vi "Check and update pretomo counters.vi"(8 "error in (no error)":errorcluster, 11 "Tomo in":refnum<class "Tomo.lvclass">) -> (0 "error out":errorcluster, 1 "continue stack?":bool, 2 "continue acquiring?":bool, 3 "Tomo out":refnum<class "Tomo.lvclass">)   [LabVIEW 2012, in "Tomo.lvclass"]
uses:
  Tomo.lvclass
  Tomo.lvclass/Tomo.ctl
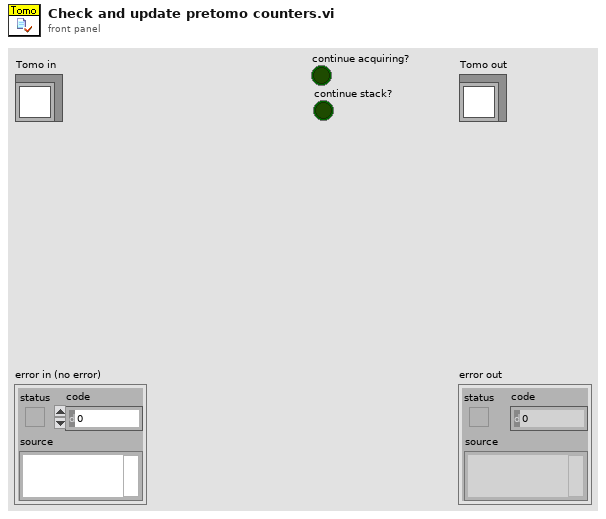
[diagram p1: front panel]
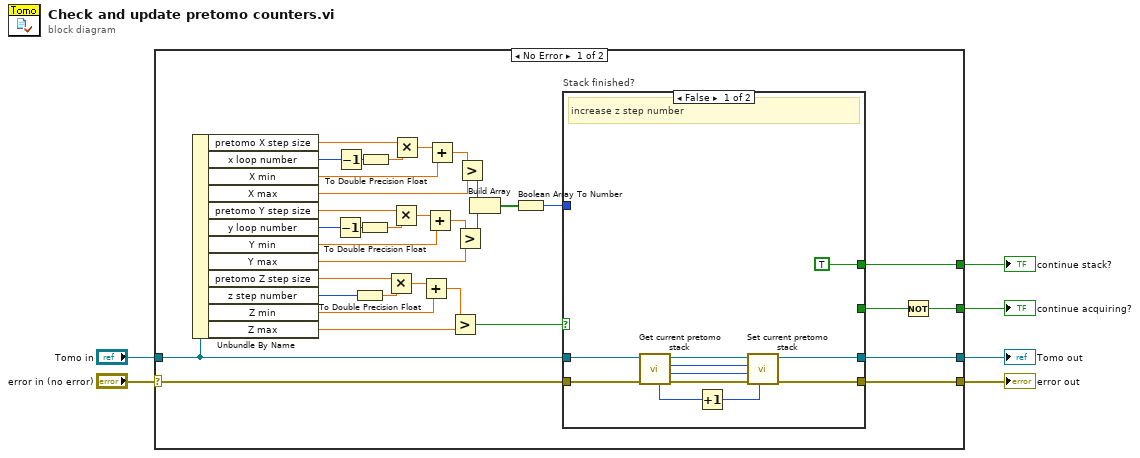
[diagram p0: block diagram]
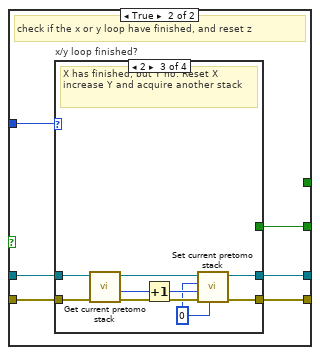
[diagram p2: hidden frame]
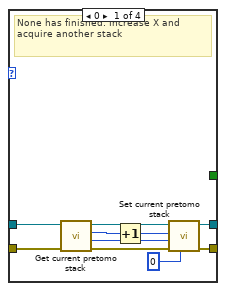
[diagram p3: hidden frame]
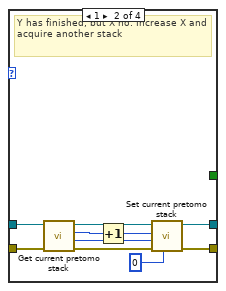
[diagram p4: hidden frame]
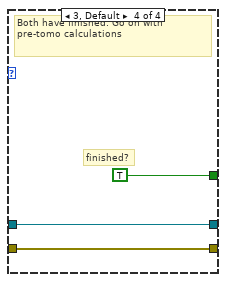
[diagram p5: hidden frame]
diagram:
  n1 = case shown="No Error" "error in (no error)" {
    selector: "error in (no error)" -> [w21 w92]
    tunnel: [w18 w92] -> w5
    tunnel: [w19 w91] -> w3
    tunnel: "Tomo in" -> [w20 w91]
    tunnel: [w16 _] -> w2
    tunnel: [w7 _] -> w1
    frame No Error {
      n2 = Unbundle By Name(w20) -> ("pretomo X step size"=w41:dbl[unit], "x loop number"=w40:i32, "X min"=w38:dbl[unit], "X max"=w35:dbl[unit], "pretomo Y step size"=w27:dbl[unit], "y loop number"=w28:i32, "Y min"=w29:dbl[unit], "Y max"=w26:dbl[unit], "pretomo Z step size"=w15:dbl[unit], "z step number"=w14:i32, "Z min"=w12:dbl[unit], "Z max"=w10:dbl[unit])
      n3 = Decrement(x=w28) -> (x-1=w31:i32)
      n4 = Decrement(x=w40) -> (x-1=w36:i32)
      n5 = To Double Precision Float(number=w14) -> (double precision float=w13:dbl)
      n6 = To Double Precision Float(number=w31) -> (double precision float=w33:dbl)
      n7 = To Double Precision Float(number=w36) -> (double precision float=w39:dbl)
      n8 = Multiply(x=w15, y=w13) -> (x*y=w11:dbl[unit])
      n9 = Multiply(x=w27, y=w33) -> (x*y=w32:dbl[unit])
      n10 = Multiply(x=w41, y=w39) -> (x*y=w37:dbl[unit])
      n11 = Add(x=w11, y=w12) -> (x+y=w9:dbl[unit])
      n12 = Add(x=w32, y=w29) -> (x+y=w30:dbl[unit])
      n13 = Add(x=w37, y=w38) -> (x+y=w34:dbl[unit])
      n14 = Greater?(x=w9, y=w10) -> (0:w8:bool)
      n15 = Greater?(x=w30, y=w26) -> (0:w24:bool)
      n16 = Greater?(x=w34, y=w35) -> (0:w25:bool)
      n17 = Build Array(w25, w24) -> (w23:bool[])
      n18 = Boolean Array To Number(Boolean array=w23) -> (number=w22:u32)
      n19 = case "Stack finished?" shown="False" w8 {
        tunnel: w22 -> [_ w58]
        tunnel: w21 -> [w49 w57]
        tunnel: w20 -> [w50 w56]
        tunnel: [w48 w55] -> w19
        tunnel: [w47 w54] -> w18
        tunnel: [_ w53] -> w17
        tunnel: [TRUE _] -> w7
        frame False {
          # "increase z step number"
          n20 = call-dynamic "Get current pretomo stack.vi"("error in (no error)"=w49, "Tomo in"=w50) -> ("error out"=w52:errorcluster, "y loop number"=w45:i32, "x loop number"=w46:i32, "Tomo out"=w51:refnum<class "Tomo.lvclass">, "z step number"=w44:i32)  [unwired: 5 in]
          n21 = Increment(x=w44) -> (x+1=w43:i32)
          n22 = call-dynamic "Set current pretomo stack.vi"("z step number"=w43, "error in (no error)"=w52, "current y stack"=w45, "current x stack"=w46, "Tomo in"=w51) -> ("error out"=w47:errorcluster, "Tomo out"=w48:refnum<class "Tomo.lvclass">)  [unwired: 5 in]
        }
        frame True {
          # "check if the x or y loop have finished, and reset z"
          n23 = case "x/y loop finished?" shown="2" w58 {
            tunnel: w57 -> [w68 w72 w84 w89]
            tunnel: w56 -> [w67 w73 w85 w90]
            tunnel: [w61 w71 w81 w90] -> w55
            tunnel: [w60 w70 w80 w89] -> w54
            tunnel: [_ _ _ TRUE] -> w53
            frame 0 {
              # "None has finished. Increase X and acquire another stack"
              n24 = call-dynamic "Get current pretomo stack.vi"("error in (no error)"=w68, "Tomo in"=w67) -> ("error out"=w65:errorcluster, "y loop number"=w62:i32, "x loop number"=w66:i32, "Tomo out"=w64:refnum<class "Tomo.lvclass">)  [unwired: 5 in, 1 out]
              n25 = Increment(x=w66) -> (x+1=w63:i32)
              n26 = call-dynamic "Set current pretomo stack.vi"("z step number"=0, "error in (no error)"=w65, "current y stack"=w62, "current x stack"=w63, "Tomo in"=w64) -> ("error out"=w60:errorcluster, "Tomo out"=w61:refnum<class "Tomo.lvclass">)  [unwired: 5 in]
            }
            frame 1 {
              # "Y has finished, but X no. Increase X and acquire another stack"
              n27 = call-dynamic "Get current pretomo stack.vi"("error in (no error)"=w72, "Tomo in"=w73) -> ("error out"=w75:errorcluster, "y loop number"=w78:i32, "x loop number"=w74:i32, "Tomo out"=w76:refnum<class "Tomo.lvclass">)  [unwired: 5 in, 1 out]
              n28 = Increment(x=w74) -> (x+1=w77:i32)
              n29 = call-dynamic "Set current pretomo stack.vi"("z step number"=0, "error in (no error)"=w75, "current y stack"=w78, "current x stack"=w77, "Tomo in"=w76) -> ("error out"=w70:errorcluster, "Tomo out"=w71:refnum<class "Tomo.lvclass">)  [unwired: 5 in]
            }
            frame 2 {
              w79 = 0 ("current x stack")
              # "X has finished, but Y no. Reset X  increase Y and acquire another stack"
              n30 = call-dynamic "Get current pretomo stack.vi"("error in (no error)"=w84, "Tomo in"=w85) -> ("error out"=w87:errorcluster, "y loop number"=w83:i32, "Tomo out"=w86:refnum<class "Tomo.lvclass">)  [unwired: 5 in, 2 out]
              n31 = Increment(x=w83) -> (x+1=w82:i32)
              n32 = call-dynamic "Set current pretomo stack.vi"("z step number"=w79, "error in (no error)"=w87, "current y stack"=w82, "current x stack"=w79, "Tomo in"=w86) -> ("error out"=w80:errorcluster, "Tomo out"=w81:refnum<class "Tomo.lvclass">)  [unwired: 5 in]
            }
            frame 3, Default {
              # "finished?"
              # "Both have finished. Go on with pre-tomo calculations"
            }
          }
        }
      }
      n33 = Not(x=w17) -> (.not. x?=w16:bool)
    }
    frame Error {
    }
  }
  "error out" <- w5
  "Tomo out" <- w3
  "continue acquiring?" <- w2
  "continue stack?" <- w1
